vi "Utility - FTP Client.vi"() -> ()   [LabVIEW 2015]
uses:
  <vilib>/FTP/NI_FTP.lvlib
panel:
  in  "error in (no error)":errorcluster caption="错误输入（无错误）"
  in  "port (21)":u16=21 caption="端口(21)"
  in  "active (T)":bool=TRUE caption="主动(T)"
  in  "file specifications":T1(array[cluster])=[{"remote path"="Config.xml", "local path"=path "c:/Config.xml", "binary"=FALSE, "data"=""}] caption="文件规范"
  out "file errors":errorcluster[](array[cluster]) caption="文件错误"
  in  "password":string="Alin@iHome301" caption="密码"
  in  "user":string="Arthur" caption="用户"
  out "error out":errorcluster caption="错误输出"
  in  "host IP":string="192.168.16.202" caption="主机IP"
  # "登陆信息"
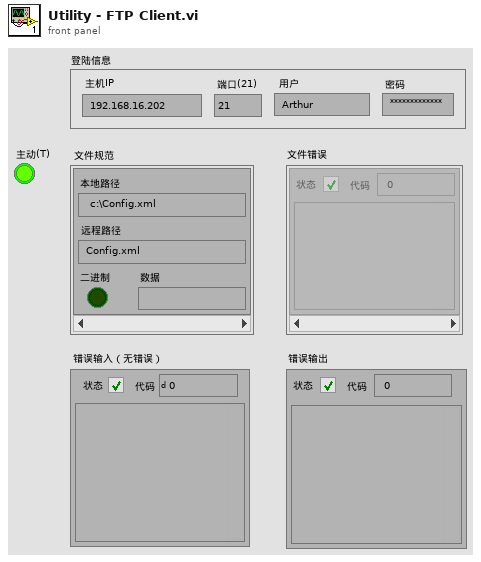
[diagram p1: front panel]
types:
  T1 = cluster{"remote path":string, "local path":path, "binary":bool, "data":string}[]
  T2 = typedef "NI_FTP.lvlib/FTP Session.ctl" = refnum<k5>
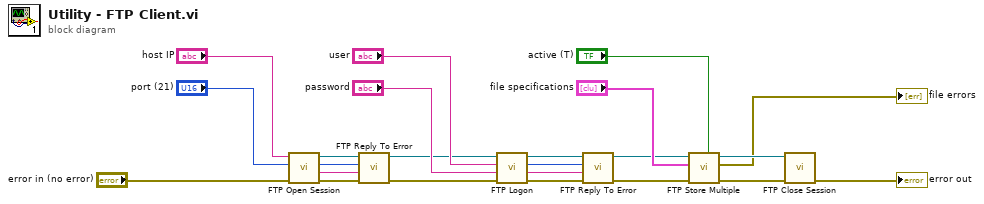
[diagram p0: block diagram]
diagram:
  n1 = call <vilib>:"FTP Open Session.vi"("error in (no error)"="error in (no error)", "remote port (21)"="port (21)", "address"="host IP") -> ("error out"=w19:errorcluster, "reply string"=w16:string, "reply code"=w17:i32, "ftp session"=w18:T2)  [unwired: 1 in, 4 out]
  n2 = call <vilib>:"FTP Reply To Error.vi"("error in (no error)"=w19, "reply string in"=w16, "reply code in"=w17, "ftp session"=w18) -> ("error out"=w14:errorcluster, "ftp session out"=w15:T2)  [unwired: 2 out]
  n3 = call <vilib>:"FTP Logon.vi"("error in (no error)"=w14, "password"="password", "user"="user", "ftp session"=w15) -> ("error out"=w13:errorcluster, "reply string"=w10:string, "reply code"=w11:i32, "ftp session out"=w12:T2)  [unwired: 4 out]
  n4 = call <vilib>:"FTP Reply To Error.vi"("error in (no error)"=w13, "reply string in"=w10, "reply code in"=w11, "ftp session"=w12) -> ("error out"=w8:errorcluster, "ftp session out"=w2:T2)  [unwired: 2 out]
  n5 = call <vilib>:"FTP Store Multiple.vi"("active (T)"="active (T)", "error in (no error)"=w8, "file specifications"="file specifications", "ftp session"=w2) -> ("error out"=w9:errorcluster, "file errors"=→"file errors":errorcluster[], "ftp session out"=w7:T2)  [unwired: 5 out]
  n6 = call <vilib>:"FTP Close Session.vi"("error in (no error)"=w9, "ftp session"=w7) -> ("error out"=→"error out":errorcluster)  [unwired: 9 out]
